vi "Set DIO Strings.vi"(7 "MISO":refnum<vi>, 8 "error in (no error)":errorcluster, 9 "Bus ref":refnum<data-value>, 10 "MOSI":refnum<vi>, 11 "ComboBox in":refnum<vi>) -> (0 "error out":errorcluster)   [LabVIEW 2014, in "Bus.lvclass"]
uses:
  Bus.lvclass
  RIO Target/RIO Target.lvclass
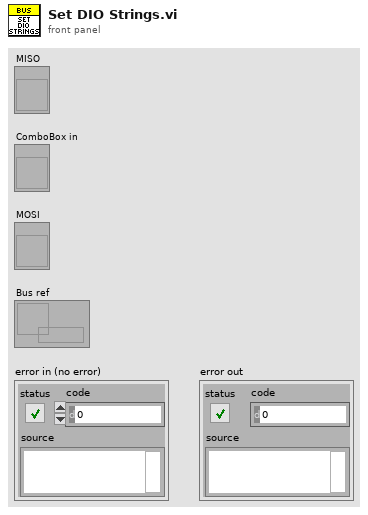
[diagram p1: front panel]
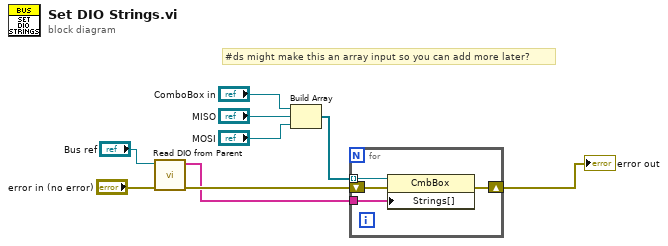
[diagram p0: block diagram]
diagram:
  # "#ds might make this an array input so you can add more later?"
  n1 = call "Read DIO from Parent.vi"("error in"="error in (no error)", "Data Value Reference in"="Bus ref") -> ("error out"=w5:errorcluster, "DIO Lines"=w2:string[])  [unwired: 8 in]
  n2 = Build Array("ComboBox in", "MISO", "MOSI") -> (w9:refnum<vi>[])
  n3 = for {
    shift-right: [w12] -> w4
    shift-left: w5 -> [w13]
    tunnel: w2 -> [w11]
    tunnel: w9 -> [w10] mode=indexing
    n4 = property class="CmbBox"(reference=w10, error in=w13, "Strings[]"=w11) -> (error out=w12:errorcluster)  [unwired: 1 out]
  }
  "error out" <- w4
